vi "Canal Plane.vi"(1 "Principal Planes":dbl[][](array[numeric]) format="%.2f") -> (0 "Canal Planes":dbl[][](array[numeric]) format="%.2f")   [LabVIEW 2013]
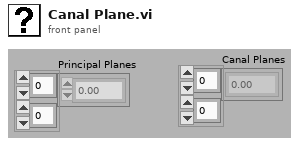
[diagram p1: front panel]
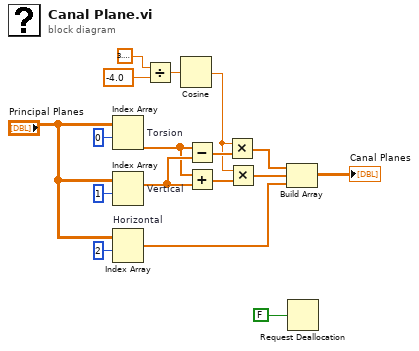
[diagram p0: block diagram]
diagram:
  n1 = Index Array "Torsion"(array="Principal Planes", index (row)=0 ("Index (row)")) -> (element=w12:dbl[])  [unwired: 1 in]
  n2 = Index Array "Vertical"(array="Principal Planes", index (row)=1 ("Index (row)")) -> (element=w13:dbl[])  [unwired: 1 in]
  n3 = Index Array "Horizontal"(array="Principal Planes", index (row)=2 ("Index (row)")) -> (element=w3:dbl[])  [unwired: 1 in]
  n4 = Divide(x=3.141592653589793, y=-4.0) -> (x/y=w9:dbl)
  n5 = Cosine(x=w9) -> (cos(x)=w6:dbl)
  n6 = Subtract(x=w12, y=w13) -> (x-y=w8:dbl[])
  n7 = Add(x=w12, y=w13) -> (x+y=w7:dbl[])
  n8 = Multiply(x=w6, y=w8) -> (x*y=w4:dbl[])
  n9 = Multiply(x=w6, y=w7) -> (x*y=w5:dbl[])
  n10 = Build Array(w4, w5, w3) -> (→"Canal Planes":dbl[][])
  n11 = Request Deallocation(FALSE ("flag")) -> ()
